vi "430_Communication_test.vi"() -> ()   [LabVIEW 2013]
panel:
  out "error out":T1
  in  "error in":T1
  in  "Y-Axis Communications Config":T2={"GPIB address"=22, "GPIB bus"=0, "connection ID"=refnum, "IP"="111.111.111.2", "Active Comm Interface"=0, "Serial Port"="", "Programmer Type"=0} {"Programmer Type" items=["Model 430", "Model 420"]; "Active Comm Interface" items=["TCP/IP (Model 430 Only)", "RS232", "IEEE488"]}
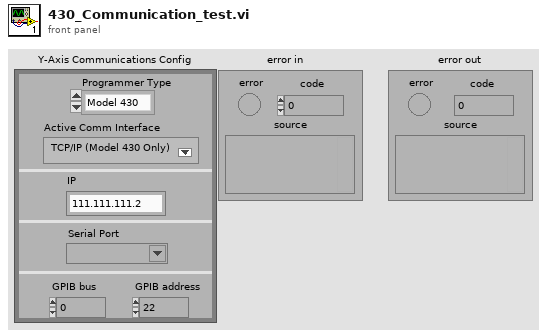
[diagram p1: front panel]
types:
  T1 = cluster{"error":bool, "code":i32, "source":string}
  T2 = cluster{"GPIB address":i16, "GPIB bus":i16, "connection ID":refnum<k5>, "IP":string, "Active Comm Interface":u16, "Serial Port":refnum<visa-resource-name>, "Programmer Type":u16}
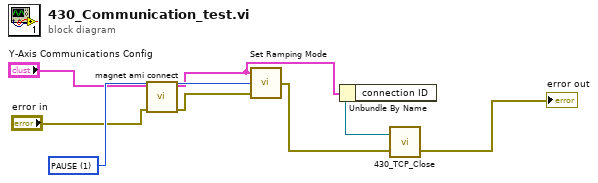
[diagram p0: block diagram]
diagram:
  w8 = u16 1 items=["RAMP", "PAUSE", "MANUAL UP", "MANUAL DOWN", "ZERO"] ("Ramping Mode")
  n1 = call "magnet ami connect.vi"("error in (no error)"="error in", "Y-Axis Communications Config"="Y-Axis Communications Config") -> ("error out"=w4:errorcluster, "Y-Axis Communications Config Out"=w3:T2)  [unwired: 7 in, 1 out]
  n2 = call <userlib>:"Set Ramping Mode.vi"("error in"=w4, "Ramping Mode"=w8, "Communications Config"=w3) -> ("error out"=w2:T1)
  n3 = Unbundle By Name(w3) -> ("connection ID"=w5:refnum<k5>)
  n4 = call <userlib>:"430_TCP_Close.vi"("error in (no error)"=w2, "connection ID"=w5) -> ("error out"=→"error out":errorcluster)  [unwired: 1 out]
